vi "BRig_Host_dataRunState_typeSelResult.vi"() -> ()   [LabVIEW 2014]
panel:
  out "output_idx":i32[](array[numeric])
  out "output_dataTS":u16[][](array[numeric])
  out "output_dataPlot":u16[][](array[numeric])
  out "output_updatePlot":bool
  in  "input_threshold_2":u16
  in  "input_threshold_1":u16
  in  "input_iSelection":u16
  in  "input_tSelection":u16
  in  "input_sSelection":u16
  in  "input_LorR":u16
  in  "input_nTrial":u16
  in  "input_idx":i32[](array[numeric])
  in  "input_dataTS":u16[][](array[numeric])
  in  "input_dataPlot":u16[][](array[numeric])
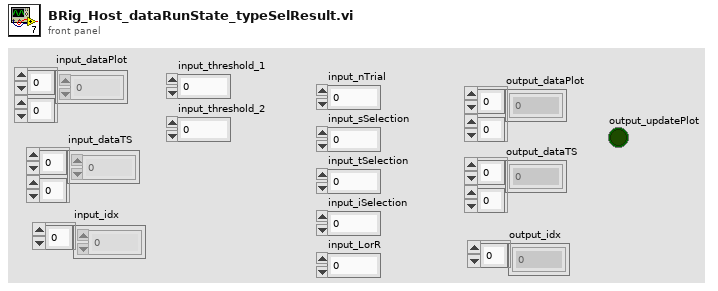
[diagram p1: front panel]
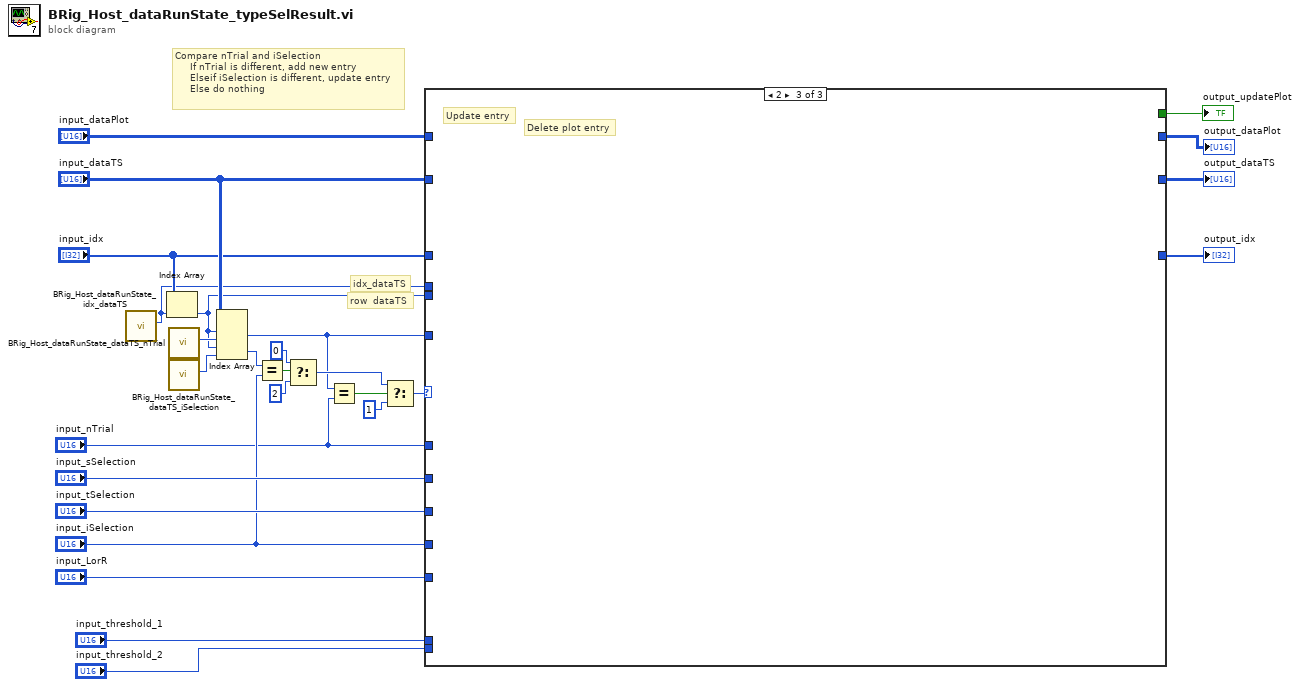
[diagram p0: block diagram]
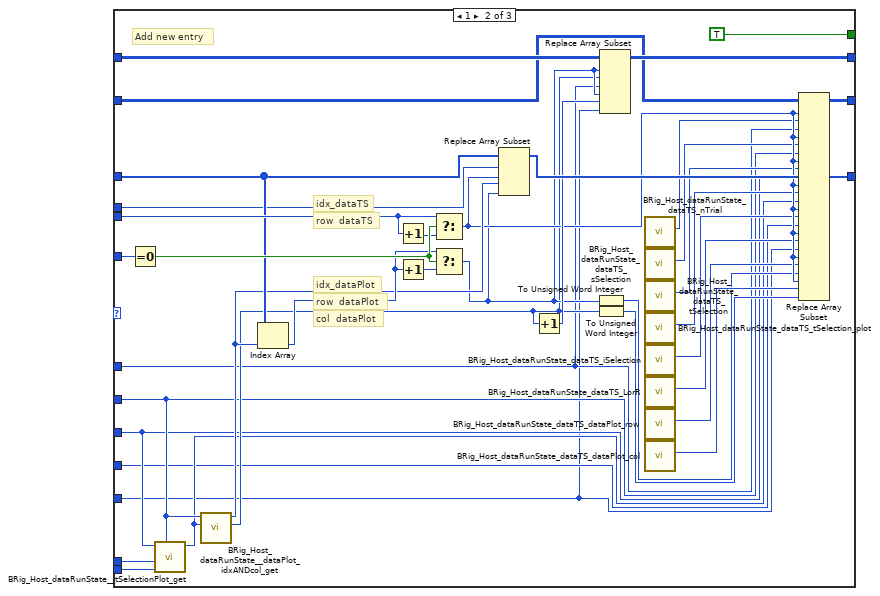
[diagram p3: hidden frame]
diagram:
  # "row  dataTS"
  # "idx_dataTS"
  # "Compare nTrial and iSelection\n     If nTrial is different, add new entry\n     Elseif iSelection is different, update entry\n     Else do nothing"
  n1 = call "BRig_Host_dataRunState_idx_dataTS.vi"() -> ("output_idx_dataTS"=w14:i32)  [unwired: 11 in]
  n2 = Index Array(array="input_idx", index=w14) -> (element=w13:i32)
  n3 = call "BRig_Host_dataRunState_dataTS_nTrial.vi"() -> ("output_idx_dataTS_nTrial"=w27:i32)  [unwired: 11 in]
  n4 = call "BRig_Host_dataRunState_dataTS_iSelection.vi"() -> ("output_idx_dataTS_iSelection"=w26:i32)  [unwired: 11 in]
  n5 = Index Array(array="input_dataTS", index (row) #1=w13, index (col) #1=w27, index (row) #2=w13, index (col) #2=w26) -> (element #1=w5:u16, element #2=w23:u16)
  n6 = Equal?(x=w23, y="input_iSelection") -> (x = y?=w22:bool)
  n7 = Select(t=u8 0, s=w22, f=u8 2) -> (s? t:f=w19:u8)
  n8 = Equal?(x=w5, y="input_nTrial") -> (x = y?=w25:bool)
  n9 = Select(t=w19, s=w25, f=u8 1) -> (s? t:f=w18:u8)
  n10 = case shown="2" w18 {
    tunnel: "input_dataPlot" -> [w30 w55 _]
    tunnel: [w30 w53 _] -> w3
    tunnel: "input_dataTS" -> [w29 w52 _]
    tunnel: [w29 w51 _] -> w2
    tunnel: "input_idx" -> [w28 w59 _]
    tunnel: [w28 w56 _] -> w1
    tunnel: w14 -> [_ w58 _]
    tunnel: w13 -> [_ w63 _]
    tunnel: "input_sSelection" -> [_ w36 _]
    tunnel: "input_tSelection" -> [_ w35 _]
    tunnel: "input_LorR" -> [_ w32 _]
    tunnel: "input_iSelection" -> [_ w33 _]
    tunnel: "input_threshold_1" -> [_ w66 _]
    tunnel: "input_threshold_2" -> [_ w67 _]
    tunnel: "input_nTrial" -> [_ w37 _]
    tunnel: w5 -> [_ w65 _]
    tunnel: [_ TRUE _] -> w4
    frame 0, Default {
      # "Do nothing"
    }
    frame 1 {
      # "col  dataPlot"
      # "row  dataPlot"
      # "idx_dataPlot"
      # "row  dataTS"
      # "idx_dataTS"
      # "Add new entry"
      n11 = Equal To 0?(x=w65) -> (x = 0?=w64:bool)
      n12 = call "BRig_Host_dataRunState__tSelectionPlot_get.vi"("input_sSelection"=w36, "input_threshold_2"=w67, "input_threshold_1"=w66, "input_tSelection"=w35) -> ("output_tSelection_plot"=w34:u16)  [unwired: 7 in]
      n13 = call "BRig_Host_dataRunState__dataPlot_idxANDcol_get.vi"("input_tSelection_plot"=w34, "input_sSelection"=w36) -> ("output_col_dataPlot"=w40:i32, "output_idx_dataPlot"=w57:i32)  [unwired: 8 in]
      n14 = Index Array(array=w59, index=w57) -> (element=w60:i32)
      n15 = Increment(x=w63) -> (x+1=w62:i32)
      n16 = Increment(x=w60) -> (x+1=w61:i32)
      n17 = Select(t=w63, s=w64, f=w62) -> (s? t:f=w50:i32)
      n18 = Select(t=w60, s=w64, f=w61) -> (s? t:f=w41:i32)
      n19 = Replace Array Subset(array=w59, new element #1=w50, index #1=w58, new element #2=w41, index #2=w57) -> (w56:i32[])
      n20 = Increment(x=w40) -> (x+1=w54:i32)
      n21 = To Unsigned Word Integer(number=w41) -> (unsigned 16bit integer=w39:u16)
      n22 = To Unsigned Word Integer(number=w40) -> (unsigned 16bit integer=w38:u16)
      n23 = Replace Array Subset(array=w55, new element #1=w37, index (row) #1=w41, index (col) #1=w40, new element #2=w32, index (row) #2=w41, index (col) #2=w54) -> (w53:u16[][])
      n24 = call "BRig_Host_dataRunState_dataTS_nTrial.vi"() -> ("output_idx_dataTS_nTrial"=w49:i32)  [unwired: 11 in]
      n25 = call "BRig_Host_dataRunState_dataTS_sSelection.vi"() -> ("output_idx_dataTS_sSelection"=w48:i32)  [unwired: 11 in]
      n26 = call "BRig_Host_dataRunState_dataTS_tSelection.vi"() -> ("output_idx_dataTS_tSelection"=w47:i32)  [unwired: 11 in]
      n27 = call "BRig_Host_dataRunState_dataTS_tSelection_plot.vi"() -> ("output_idx_dataTS_tSelection_plot"=w46:i32)  [unwired: 11 in]
      n28 = call "BRig_Host_dataRunState_dataTS_iSelection.vi"() -> ("output_idx_dataTS_iSelection"=w45:i32)  [unwired: 11 in]
      n29 = call "BRig_Host_dataRunState_dataTS_LorR.vi"() -> ("output_idx_dataTS_LorR"=w44:i32)  [unwired: 11 in]
      n30 = call "BRig_Host_dataRunState_dataTS_dataPlot_row.vi"() -> ("output_idx_dataTS_dataPlot_row"=w43:i32)  [unwired: 11 in]
      n31 = call "BRig_Host_dataRunState_dataTS_dataPlot_col.vi"() -> ("output_idx_dataTS_dataPlot_col"=w42:i32)  [unwired: 11 in]
      n32 = Replace Array Subset(array=w52, new element #1=w37, index (row) #1=w50, index (col) #1=w49, new element #2=w36, index (row) #2=w50, index (col) #2=w48, new element #3=w35, index (row) #3=w50, index (col) #3=w47, new element #4=w34, index (row) #4=w50, index (col) #4=w46, new element #5=w33, index (row) #5=w50, index (col) #5=w45, new element #6=w32, index (row) #6=w50, index (col) #6=w44, new element #7=w39, index (row) #7=w50, index (col) #7=w43, new element #8=w38, index (row) #8=w50, index (col) #8=w42) -> (w51:u16[][])
    }
    frame 2 {
      # "Delete plot entry"
      # "Update entry"
    }
  }
  "output_updatePlot" <- w4
  "output_dataPlot" <- w3
  "output_dataTS" <- w2
  "output_idx" <- w1
